vi "Main_009.vi"() -> ()   [LabVIEW 2025]
uses:
  Utility/Universal Utility/TypeDefs_Utility/Cluster_Row-Column.ctl
  9e3f57c0-2ef8-4495-8287-c6a42a5fb955.vi
  Utility/Universal Utility/TypeDefs_Utility/ENUM_4 Directions U-D-L-R.ctl
  Utility/Universal Utility/TypeDefs_Utility/ENUM_8 Directions U-D-L-R.ctl
panel:
  out "Product":u64[](array[numeric])
  out "Sum":u64[](array[numeric])
  out "Array":u64[][](array[numeric])
  out "squares":u64[](array[numeric])
  out "nums":u64[](array[numeric])
  out "MATCH":bool
  in  "Select Data":enum32{"Example", "Puzzle"}(tab)
  in  "EX Target":u64=60
  in  "Example Input":u64=17
  in  "Puzzle Input":u64=1000
  in  "Puzzle Target":u64=31875000
  out "Answer":u64
  # "3*4*5 =60"
  # "3+4+5 =17"
  # "3*4*5 =60"
  # "a+b+c=1000"
  # "a*b*c=X"
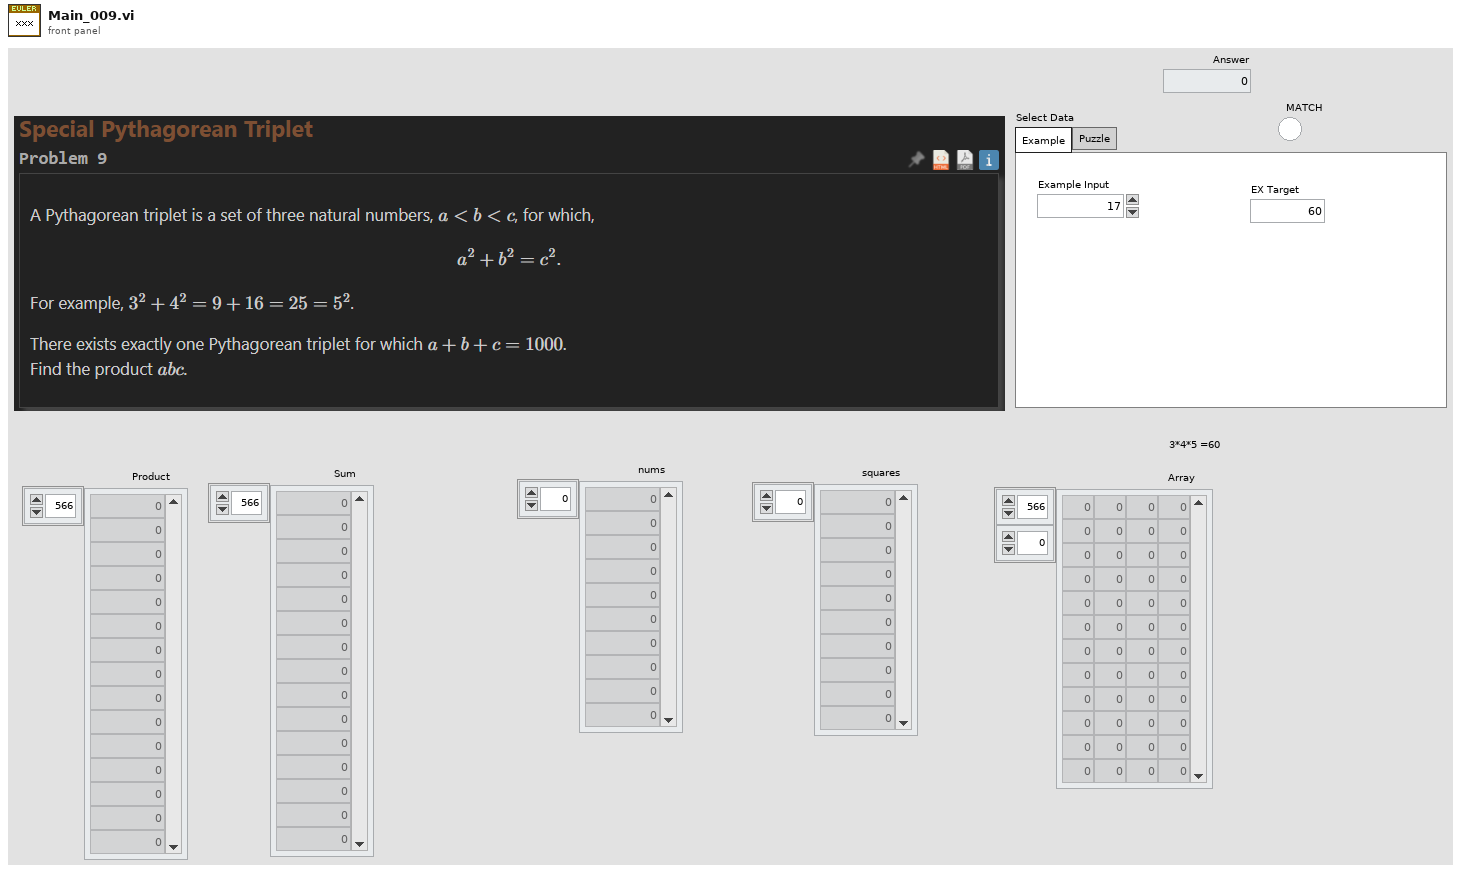
[diagram p1: front panel]
types:
  T1 = typedef "ENUM_8 Directions U-D-L-R.ctl" = enum16{"Up;-1,0", "Up-Right;-1,1", "Right;0,1", "Down-Right;1,1", "Down;1,0", "Down-Left;1,-1", "Left;0,-1", "Up-Left;-1,-1"}
  T2 = typedef "ENUM_4 Directions U-D-L-R.ctl" = enum16{"Up;-1,0", "Right;0,1", "Down;1,0", "Left;0,-1"}
  T3 = typedef "Cluster_Row-Column.ctl" = cluster{"R":i32, "C":i32}
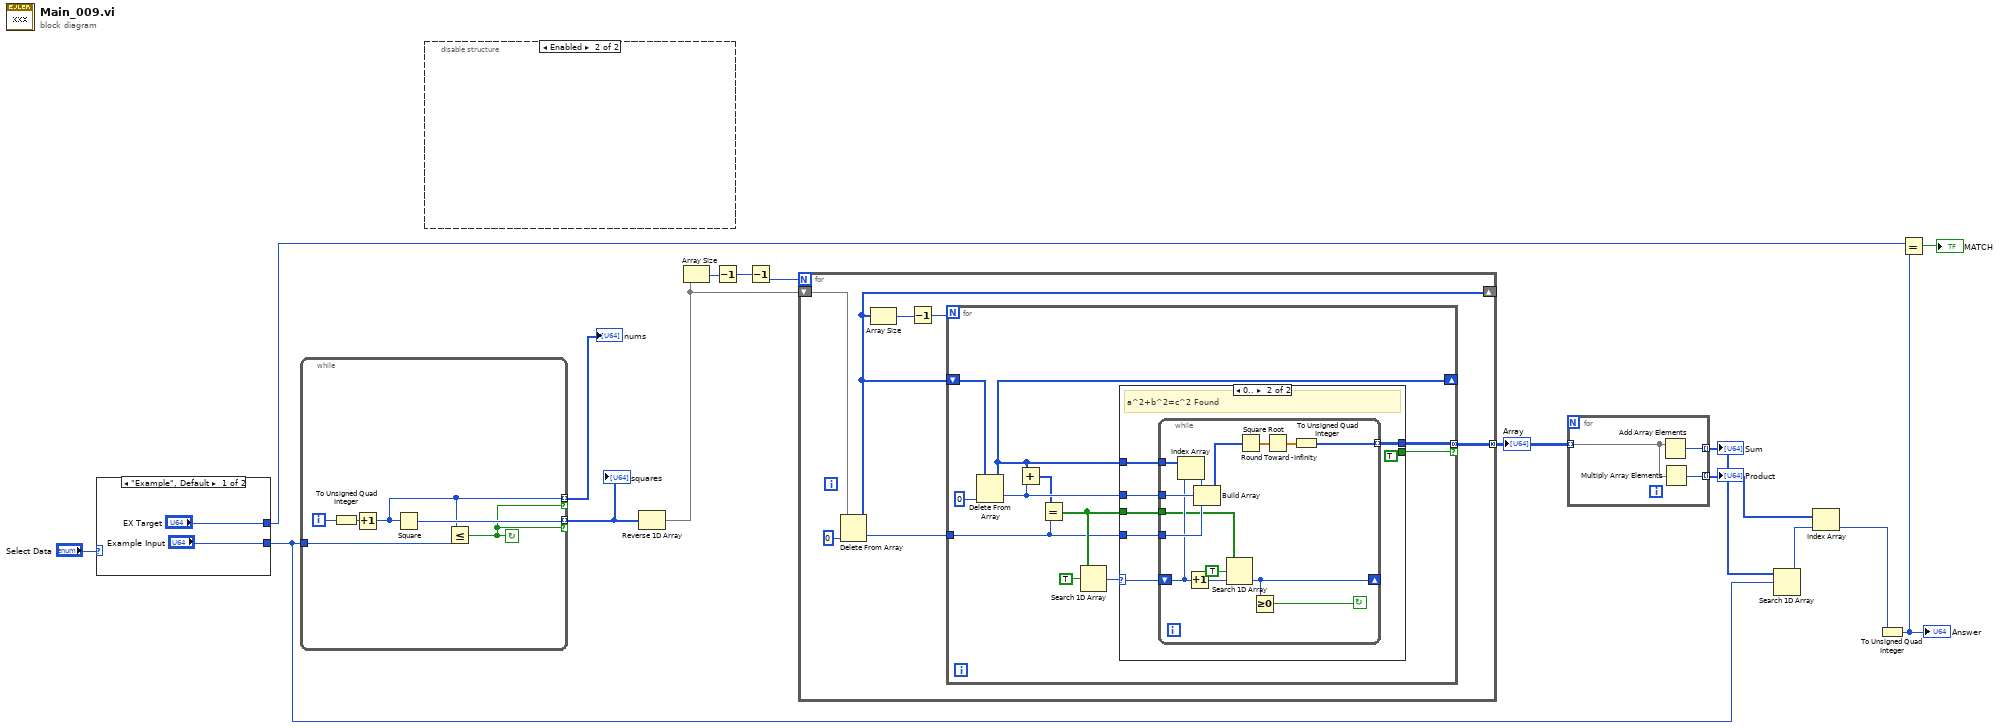
[diagram p0: block diagram]
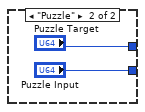
[diagram p3: hidden frame]
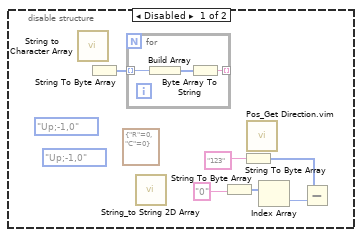
[diagram p4: hidden frame]
diagram:
  n1 = case shown="\"Example\", Default" "Select Data" {
    tunnel: ["Example Input" "Puzzle Input"] -> w4
    tunnel: ["EX Target" "Puzzle Target"] -> w14
    frame "Example", Default {
    }
    frame "Puzzle" {
    }
  }
  n2 = while {
    tunnel: w4 -> [w24]
    tunnel: [w25] -> w11 mode=indexing if=w22
    tunnel: [w21] -> w12 mode=indexing if=w22
    i -> [w26]
    stop <- w22 continue-if-true
    n3 = To Unsigned Quad Integer(1:w26) -> (0:w23:u64)
    n4 = Increment(x=w23) -> (x+1=w21:u64)
    n5 = Square(x=w21) -> (x^2=w25:u64)
    n6 = Less Or Equal?(x=w21, y=w24) -> (x <= y?=w22:bool)
  }
  "nums" <- w12
  "squares" <- w11
  n7 = disable-structure shown="Enabled" {
    frame Disabled {
      (unwired) ENUM_8_Directions_U-D-L-R."Up;-1,0" ("Direction 8")
      (unwired) ENUM_4_Directions_U-D-L-R."Up;-1,0" ("Direction")
      (unwired) T3 {"R"=0, "C"=0} ("Position")
      n8 = call "String to Character Array.vi"() -> ()  [unwired: 1 in, 1 out]
      n9 = String To Byte Array() -> (unsigned byte array=w27:u8[])  [unwired: 1 in]
      n10 = for {
        tunnel: w27 -> [w35] mode=indexing
        tunnel: [w33] -> _ mode=indexing
        n11 = Build Array(w35) -> (w34:u8[])
        n12 = Byte Array To String(unsigned byte array=w34) -> (string=w33:string)
      }
      n13 = call "String_to String 2D Array.vi"() -> ()  [unwired: 11 in, 1 out]
      n14 = String To Byte Array(string="0") -> (unsigned byte array=w30:u8[])
      n15 = String To Byte Array(string="123") -> (unsigned byte array=w28:u8[])
      n16 = call "Pos_Get Direction.vim"() -> ()  [unwired: 11 in, 1 out]
      n17 = Index Array(array=w30) -> (element=w29:u8)  [unwired: 1 in]
      n18 = Subtract(x=w28, y=w29) -> ()  [unwired: 1 out]
    }
    frame Enabled {
    }
  }
  n19 = Reverse 1D Array(array=w11) -> (reversed array=w10:u64[])
  n20 = Array Size(array=w10) -> (size(s)=w9:i32)
  n21 = Decrement(x=w9) -> (x-1=w8:i32)
  n22 = Decrement(x=w8) -> (x-1=w7:i32)
  n23 = for {
    N: w7 -> [_]
    shift-right: [w38] -> _
    shift-left: w10 -> [w42]
    tunnel: [w39] -> w6 mode=concatenating
    n24 = Delete From Array(array=w42, index=0) -> (deleted portion=w40:u64, array with subset deleted=w38:u64[])  [unwired: 1 in]
    n25 = Array Size(array=w38) -> (size(s)=w37:i32)
    n26 = Decrement(x=w37) -> (x-1=w36:i32)
    n27 = for {
      N: w36 -> [_]
      shift-right: [w44] -> _
      shift-left: w38 -> [w53]
      tunnel: w40 -> [w48]
      tunnel: [w46] -> w39 mode=concatenating if=w45
      n28 = Delete From Array(array=w53, index=0) -> (deleted portion=w47:u64, array with subset deleted=w44:u64[])  [unwired: 1 in]
      n29 = Add(x=w44, y=w47) -> (x+y=w43:u64[])
      n30 = Equal?(x=w43, y=w48) -> (x = y?=w49:bool[])
      n31 = Search 1D Array(1D array=w49, element=TRUE) -> (index of element=w50:i32)  [unwired: 1 in]
      n32 = case shown="0.." w50 {
        selector: w50 -> [_ w60]
        tunnel: w49 -> [_ w59]
        tunnel: w44 -> [_ w56]
        tunnel: w48 -> [_ w58]
        tunnel: w47 -> [_ w57]
        tunnel: [_ w55] -> w46
        tunnel: [_ TRUE] -> w45
        frame ..-1 {
          # "a^2+b^2=c^2 NOT Found"
        }
        frame 0.. {
          # "a^2+b^2=c^2 Found"
          n33 = while {
            shift-right: [w65] -> _
            shift-left: w60 -> [w69]
            tunnel: w59 -> [w68]
            tunnel: w58 -> [w71]
            tunnel: w57 -> [w72]
            tunnel: w56 -> [w74]
            tunnel: [w61] -> w55 mode=indexing
            stop <- w64 continue-if-true
            n34 = Index Array(array=w74, index=w69) -> (element=w73:u64)
            n35 = Increment(x=w69) -> (x+1=w67:i32)
            n36 = Build Array(w73, w72, w71) -> (w70:u64[])
            n37 = Search 1D Array(1D array=w68, element=TRUE, start index (0)=w67) -> (index of element=w65:i32)
            n38 = Square Root(x=w70) -> (sqrt(x)=w63:dbl[])
            n39 = Greater Or Equal To 0?(x=w65) -> (x >= 0?=w64:bool)
            n40 = Round Toward -Infinity(1:w63) -> (0:w62:dbl[])
            n41 = To Unsigned Quad Integer(1:w62) -> (0:w61:u64[])
          }
        }
      }
    }
  }
  "Array" <- w6
  n42 = for {
    tunnel: w6 -> [w77] mode=indexing
    tunnel: [w76] -> w5 mode=indexing
    tunnel: [w75] -> w3 mode=indexing
    n43 = Add Array Elements(numeric array=w77) -> (sum=w76:u64)
    n44 = Multiply Array Elements(1:w77) -> (0:w75:u64)
  }
  "Sum" <- w5
  "Product" <- w3
  n45 = Search 1D Array(1D array=w5, element=w4) -> (index of element=w2:i32)  [unwired: 1 in]
  n46 = Index Array(array=w3, index=w2) -> (element=w1:u64)
  n47 = To Unsigned Quad Integer(1:w1) -> (0:w13:u64)
  "Answer" <- w13
  n48 = Equal?(x=w14, y=w13) -> (x = y?=→"MATCH":bool)
